vi "Read Local Port.vi"(11 "TCP Stream in":refnum<class "TCP Stream.lvclass">) -> (2 "local port":u16=2001)   [LabVIEW 2020, in "TCP Stream.lvclass"]
doc: "Returns the local IP port being used by this stream connection."
uses:
  TCP Stream.lvclass
  TCP Stream.lvclass/TCP Stream.ctl
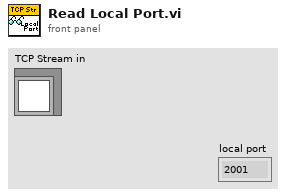
[diagram p1: front panel]
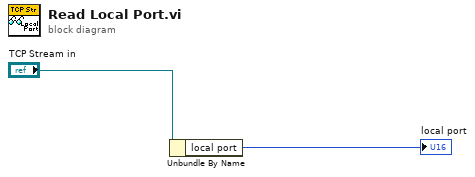
[diagram p0: block diagram]
diagram:
  n1 = Unbundle By Name("TCP Stream in") -> ("local port"=→"local port":u16)
